vi "Scan Engine GUIDs.vi"() -> ()   [LabVIEW 2016, in "Scan Engine Custom Device.lvlib"]
uses:
  Scan Engine Custom Device.lvlib
panel:
  in  "EtherCAT 9145 Slave":string="F08D8E42-E070-4D6E-B502-45A5BF0753B8"
  in  "EtherCAT 9144 Slave":string="0967D9B5-C270-4E7D-AF0D-EBA564935FF3"
  in  "Scan Engine Main Disabled":string="648dbacc-166f-4d11-a145-bec5ccc39f70"
  in  "Scan Engine Custom Main IO Network Variables":string="0ED332F0-D1BC-432A-B546-E056CE863643"
  in  "ECAT I/O Network Variables":string="385C8ABA-3B7C-4183-A2E4-B1B8A7B2DFC9"
  in  "EtherCAT Generic  Slave":string="79b01192-925a-419a-aca0-9b5b4a565a1e"
  in  "Slot - Empty":string="41F294B5-009B-733F-41B9-7972E3D57FD3"
  in  "Slot - Disabled":string="C37AE504-7B62-8355-1600-C9D1A9C81815"
  in  "From FPGA Channel - Digital":string="B0022617-ACA6-3A27-F901-F70AB50C6C00"
  in  "To FPGA Channel - Digital":string="21A3511E-B5B7-DAD1-9B8C-1391802D6061"
  in  "From FPGA Channel - Unsupported":string="C8197AFD-3C01-E731-6DE4-E2ECB7F7C6AF"
  in  "To FPGA Channel - Unsupported":string="492D2E26-3388-59A7-4A05-53B4509008DB"
  in  "User Vars Page - ECAT":string="A16C5AEF-BF42-EF6D-BC81-FD52AB4F64C4"
  in  "EtherCAT Master":string="207C3DCA-1177-DD2C-D32C-1F1D46E93318"
  in  "Local Chassis":string="E829C44F-D204-78F7-F536-2C86E8FAC5FB"
  in  "TC Channel":string="2D047D7F-FAEE-AA5E-DB50-5E1C690ADDE7"
  in  "From FPGA Channel - Analog":string="725DE6B0-41A1-A0E4-E2CD-A132E5FCC5EA"
  in  "To FPGA Channel - Analog":string="08CD8252-70E6-0957-DDD7-77D59D7DC2E9"
  in  "User Vars Page - Local":string="0244C2CA-486B-E148-C1E2-82323B844A49"
  in  "EtherCAT 914x Slave":string="50877E70-98F5-BFCC-3809-88209D9D28F5"
  in  "Slot":string="A466E035-6C67-FF94-A582-AF548F5C2F28"
  in  "Scan Engine Main Page":string="A04A67D4-9B64-052B-A031-6B05377B9B10"
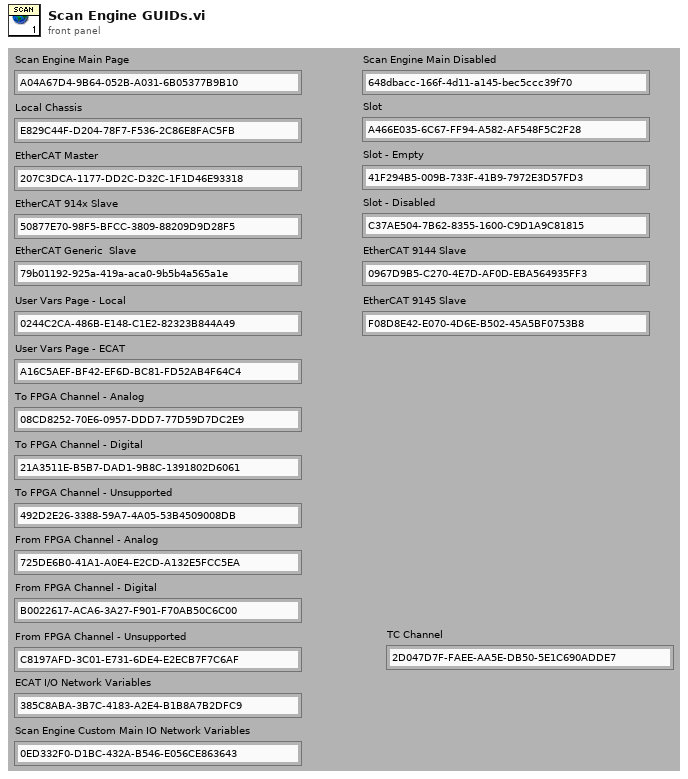
[diagram p1: front panel]
diagram:
